vi "Read Measurement (Edge).vi"(0 "VISA resource name":refnum<visa-resource-name>, 9 "Maximum Time (10000ms)":u32=10000, 11 "error in (no error)":errorcluster) -> (4 "VISA resource name out":refnum<visa-resource-name>, 6 "Edge Time":dbl, 15 "error out":errorcluster)   [LabVIEW 2020, in "Agilent 90000 Series.lvlib"]
doc: "Measures the time of the edge, relative to the reference location.\n\nThis VI initiates an acquisition on the channel that the end-user defines. It then waits for the acquisition to complete, obtains a waveform measurement on the channel the end-user specifies, and returns the measurement value."
uses:
  Agilent 90000 Series.lvlib
  Low Level/Fetch Measurement (Edge).vi
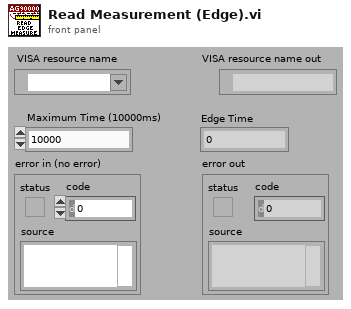
[diagram p1: front panel]
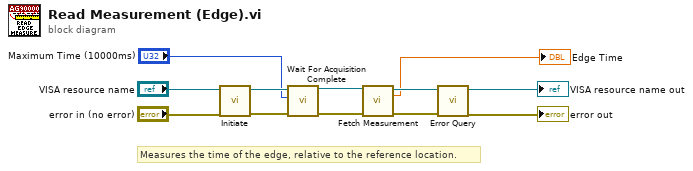
[diagram p0: block diagram]
diagram:
  # "Measures the time of the edge, relative to the reference location."
  n1 = call "Initiate.vi"("error in (no error)"="error in (no error)", "VISA resource name"="VISA resource name") -> ("error out"=w10:errorcluster, "VISA resource name out"=w9:refnum<visa-resource-name>)  [unwired: 8 out]
  n2 = call "Wait For Acquisition Complete.vi"("error in (no error)"=w10, "Maximum Time (10000ms)"="Maximum Time (10000ms)", "VISA resource name"=w9) -> ("error out"=w4:errorcluster, "VISA resource name out"=w5:refnum<visa-resource-name>)  [unwired: 7 out]
  n3 = call-poly "Fetch Measurement.vi"("VISA resource name"=w5, "error in (no error)"=w4) -> ("VISA resource name out"=w3:refnum<visa-resource-name>, "Edge Time"=→"Edge Time":dbl, "error out"=w2:errorcluster)  [unwired: 11 out]
  n4 = call "Error Query.vi"("error in (no error)"=w2, "VISA resource name"=w3) -> ("error out"=→"error out":errorcluster, "VISA resource name out"=→"VISA resource name out":refnum<visa-resource-name>)  [unwired: 8 out]
